vi "Set Default Ref Clock Source.vi"(8 "error in (no error)":errorcluster, 10 "Default Reference Source (T: Internal)":bool=TRUE, 11 "VISA resource name":refnum<visa-resource-name>) -> (0 "error out":errorcluster, 3 "VISA resource name out":refnum<visa-resource-name>)   [LabVIEW 2013, in "Fluke 5XXX Series Multicalibrators.lvlib"]
doc: "This VI sets the power-up and reset default for the reference clock source (internal or through the 10 MHz IN BNC connector).\n\nNote:\n\nThis VI is available only for instrument model 5520A."
uses:
  Fluke 5XXX Series Multicalibrators.lvlib
panel:
  # "Internal"
  # "External"
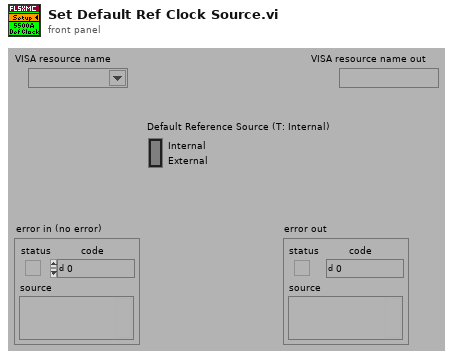
[diagram p1: front panel]
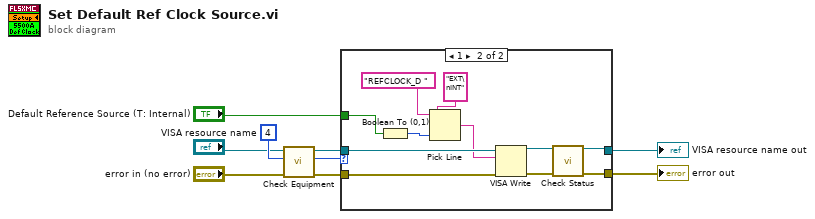
[diagram p0: block diagram]
diagram:
  n1 = call "Check Equipment.vi"("error in (no error)"="error in (no error)", "Bit Mask"=4 ("Numeric"), "VISA resource name"="VISA resource name") -> ("error out"=w8:errorcluster, "Present?"=w7:u32, "VISA resource name out"=w6:refnum<visa-resource-name>)  [unwired: 6 in]
  n2 = case shown="1" w7 {
    tunnel: "Default Reference Source (T: Internal)" -> [_ w19]
    tunnel: [w10 w14] -> w2
    tunnel: w8 -> [w11 w18]
    tunnel: w6 -> [w10 w17]
    tunnel: [w11 w15] -> w3
    frame 0, Default {
    }
    frame 1 {
      n3 = Boolean To (0,1)(Boolean=w19) -> (0, 1=w20:i16)
      n4 = Pick Line(string ("")="REFCLOCK_D " ("Reset Command"), multi-line string="EXT\nINT", line index=w20) -> (output string=w16:string)
      n5 = VISA Write(VISA resource name=w17, write buffer=w16, error in (no error)=w18) -> (VISA resource name out=w13:refnum<visa-resource-name>, error out=w12:errorcluster)  [unwired: 1 out]
      n6 = call "Check Status.vi"("VISA resource name"=w13, "error in (no error)"=w12) -> ("VISA resource name out"=w14:refnum<visa-resource-name>, "error out"=w15:errorcluster)  [unwired: 12 in]
    }
  }
  "VISA resource name out" <- w2
  "error out" <- w3
